vi "save_to_15min.vi"(11 "error_code":i32) -> ()   [LabVIEW 2018]
uses:
  <vilib>/Utility/file.llb/Write Delimited Spreadsheet (DBL).vi
  Labview/SeaBreeze.lvlib
panel:
  out "XY图":cluster{dbl[], "buffer out":dbl[]}(graph)
  out "数值":i32
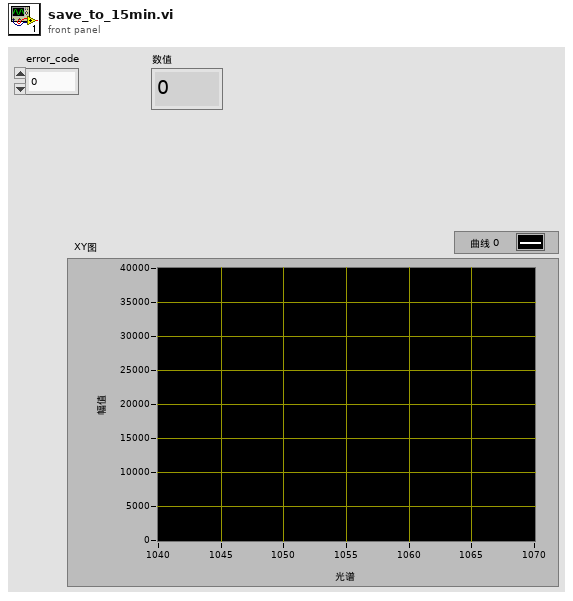
[diagram p1: front panel]
types:
  T1 = cluster{"wavelengths out":dbl[], "buffer out":dbl[]}
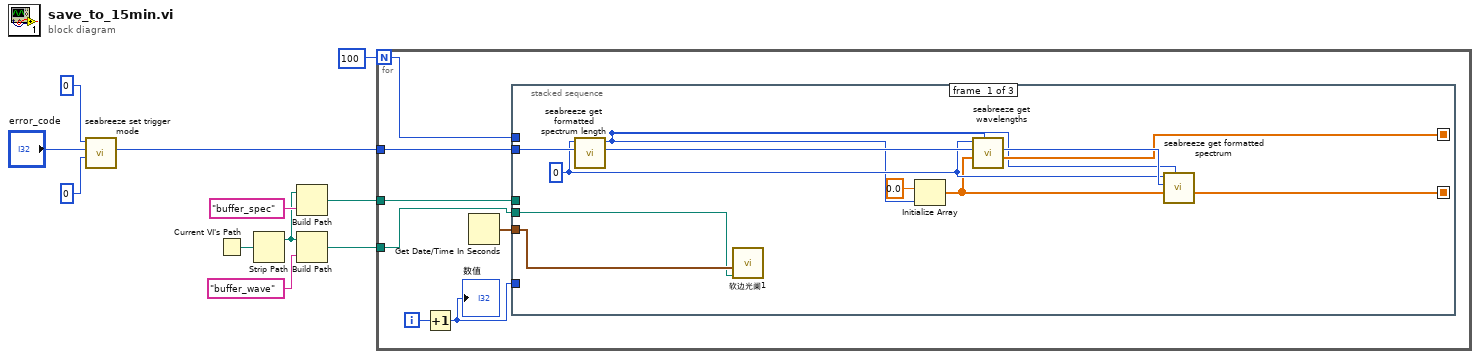
[diagram p0: block diagram]
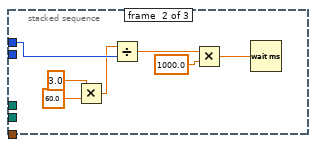
[diagram p2: hidden frame]
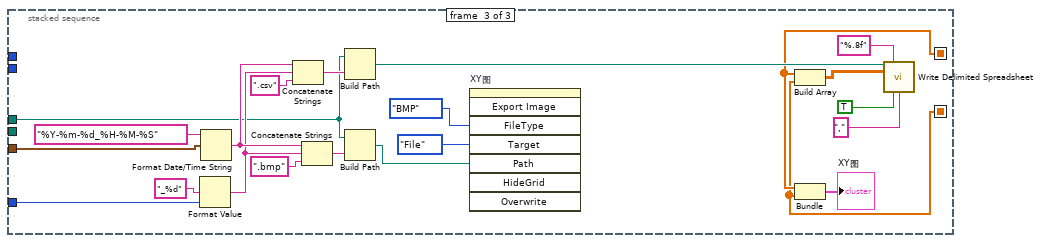
[diagram p3: hidden frame]
diagram:
  n1 = call "seabreeze set trigger mode.vi"("mode"=0, "error_code"="error_code", "index"=0) -> ("error_code out"=w7:i32)  [unwired: 8 in]
  n2 = Current VI's Path() -> (path=w11:path)
  n3 = Strip Path(path=w11) -> (stripped path=w4:path)  [unwired: 1 out]
  n4 = Build Path(base path=w4, name or relative path="buffer_spec" ("名称或相对路径")) -> (appended path=w5:path)
  n5 = Build Path(base path=w4, name or relative path="buffer_wave" ("名称或相对路径")) -> (appended path=w2:path)
  n6 = for {
    N: 100 -> [w17]
    tunnel: w7 -> [w18]
    tunnel: w5 -> [w16]
    tunnel: w2 -> [w13]
    i -> [w15]
    n7 = Increment(x=w15) -> (x+1=w12:i32)
    "数值" <- w12
    n8 = Get Date/Time In Seconds() -> (seconds since 1Jan1904=w14:timestamp)
    n9 = stacked-sequence {
      seq-local: [w24 _ _] -> [_ _ w46]
      seq-local: [w23 _ _] -> [_ _ w47]
      tunnel: w18 -> [w29 _ _]
      tunnel: w17 -> [_ w36 _]
      tunnel: w16 -> [_ _ w38]
      tunnel: w12 -> [_ _ w50]
      tunnel: w14 -> [w20 _ w48]
      tunnel: w13 -> [w19 _ _]
      frame #0 {
        w26 = 0
        n10 = call "seabreeze get formatted spectrum length.vi"("error_code"=w29, "index"=w26) -> ("error_code out"=w28:i32, "function return"=w21:i32)  [unwired: 8 in]
        n11 = call "软边光阑1.vi"("Path"=w19, "time"=w20) -> ()  [unwired: 3 in, 1 out]
        n12 = Initialize Array(0.0 ("element"), w21) -> (w22:dbl[])
        n13 = call "seabreeze get wavelengths.vi"("length"=w21, "wavelengths"=w22, "error_code"=w28, "index"=w26) -> ("wavelengths out"=w23:dbl[], "error_code out"=w27:i32)  [unwired: 5 in, 1 out]
        n14 = call "seabreeze get formatted spectrum.vi"("buffer_length"=w21, "buffer"=w22, "error_code"=w27, "index"=w26) -> ("buffer out"=w24:dbl[])  [unwired: 5 in, 2 out]
      }
      frame #1 {
        n15 = Multiply(x=3.0, y=60.0) -> (x*y=w32:dbl)
        n16 = Divide(x=w32, y=w36) -> (x/y=w35:dbl)
        n17 = Multiply(x=w35, y=1000.0) -> (x*y=w34:dbl)
        n18 = Wait (ms)(milliseconds to wait=w34) -> ()  [unwired: 1 out]
      }
      frame #2 {
        n19 = Format Value(format string="_%d" ("格式字符串"), value (0)=w50) -> (output string=w41:string)  [unwired: 1 in]
        n20 = Format Date/Time String(time format string (%c)="%Y-%m-%d_%H-%M-%S" ("时间格式字符串(%c)"), seconds (now)=w48) -> (date/time string=w42:string)  [unwired: 1 in]
        n21 = Concatenate Strings(w42, w41, ".csv" ("字符串")) -> (w56:string)
        n22 = Concatenate Strings(w42, w41, ".bmp" ("字符串")) -> (w37:string)
        n23 = Build Path(base path=w38, name or relative path=w56) -> (appended path=w55:path)
        n24 = Build Path(base path=w38, name or relative path=w37) -> (appended path=w39:path)
        n25 = invoke on="XY图" class="XYGraph (严格)" method="Export Image"("FileType"=enum32{"BMP", "EPS", "EMF", "PICT"}."BMP" ("文件类型"), "Target"=enum32{"File", "Clipboard"}."File" ("目标"), "Path"=w39) -> ()  [unwired: 5 in, 8 out]
        n26 = Build Array(w47, w46) -> (w54:dbl[][])
        n27 = Bundle("wavelengths out"=w47, "buffer out"=w46) -> (→"XY图":T1)  [unwired: 1 in]
        n28 = call-poly <vilib>:"Write Delimited Spreadsheet.vi"("file path (dialog if empty)"=w55, "format (%.3f)"="%.8f", "2D data"=w54, "transpose? (no:F)"=TRUE, "delimiter (\\t)"="," ("delimiter (\\t)")) -> ()  [unwired: 9 in, 2 out]
      }
    }
  }
